vi "Get Service Class Instances.vi"() -> (3 "service instances":refnum<class "ServiceBase.lvclass">[](array[class]))   [LabVIEW 2021, in "Unary_server.lvlib"]
uses:
  Unary_server.lvlib
  <vilib>/gRPC/LabVIEW gRPC Servicer/ServiceBase/ServiceBase.lvclass
  RPC Service/I2C/I2C.lvclass
  C:/Program Files/National Instruments/LabVIEW 2021/vi.lib/gRPC/LabVIEW gRPC Servicer/ServiceBase/ServiceBase.lvclass
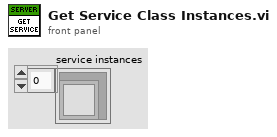
[diagram p1: front panel]
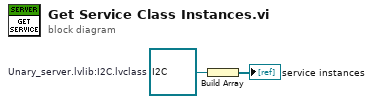
[diagram p0: block diagram]
diagram:
  w1 = refnum<class "I2C.lvclass"> refnum  # Unary_server.lvlib:I2C.lvclass
  n1 = Build Array(w1) -> (→"service instances":refnum<class "I2C.lvclass">[])
